vi "Galobal variable_TI.vi"() -> ()   [LabVIEW 2015]
panel:
  in  "Operator ID":string="OB"
  in  "Server":bool
  in  "Shift":T1
  in  "Rework bit":bool
  in  "NG Count":u8
  in  "Shift  Change":string
  in  "User ID":string="OB"
  out "Emergency Analog":bool
  out "Errror For Color":bool
  in  "Pokayoka Status":bool
  in  "Rpt Write 2":bool
  in  "Rpt Write":bool
  in  "Rpt Read":bool
  in  "Model triger":bool
  in  "Camera Bit":string
  out "Error Color":u32
  in  "Cali data":T2
  out "Camera NG":bool
  in  "CAMERA TRIGGER":bool
  out "Camera OK":bool
  out "Cordinate":string
  in  "LCD  Barcode_Trigger":bool
  in  "MIC Barcode _Trigger":bool
  in  "MIC Barcode":string
  in  "LCD Barcode":string
  in  "Barcode Setting":T3={"MIC "="", "baud rate MIC "=9600, "LCD "="COM5", "baud rate_LCD"=115200}
  out "IL Sensor_Pokayoka":bool[](array[boolean])
  in  "Running Model":string
  in  "Sensor Setting Data":T4
  out "Sensor Data":T5
  in  "NI Comm.Error":bool
  in  "LVDT":dbl format="%0.03f"
  in  "Load Cell":dbl format="%0.03f"
  in  "Digital Output":bool[](array[boolean])
  in  "Auto Exit":bool
  in  "Slid Servo Home bit":bool
  in  "Call Home M2":bool
  in  "Call Home M1":bool
  in  "Barcode Lenght":i32
  in  "Barcode Scan Bit":bool
  in  "Barcode Data":string
  in  "Control Enable":bool
  in  "Stop M1":bool
  in  "Stop M2":bool
  in  "Programlist":string[](array[string])
  in  "STM Done Bit":bool
  in  "Offset_2":dbl
  in  "Offset_1":dbl
  in  "Slop _2":dbl
  in  "Slop_1":dbl
  out "Analoge Input":dbl[](array[numeric])
  out "AI_as DI":bool[](array[boolean])
  out "Manual DO":bool[](array[boolean])
  in  "Manual CMD":bool
  out "File Path":path[](array[path])
  out "Digital input":bool[](array[boolean])
  in  "User Name":string
  in  "Exit":bool
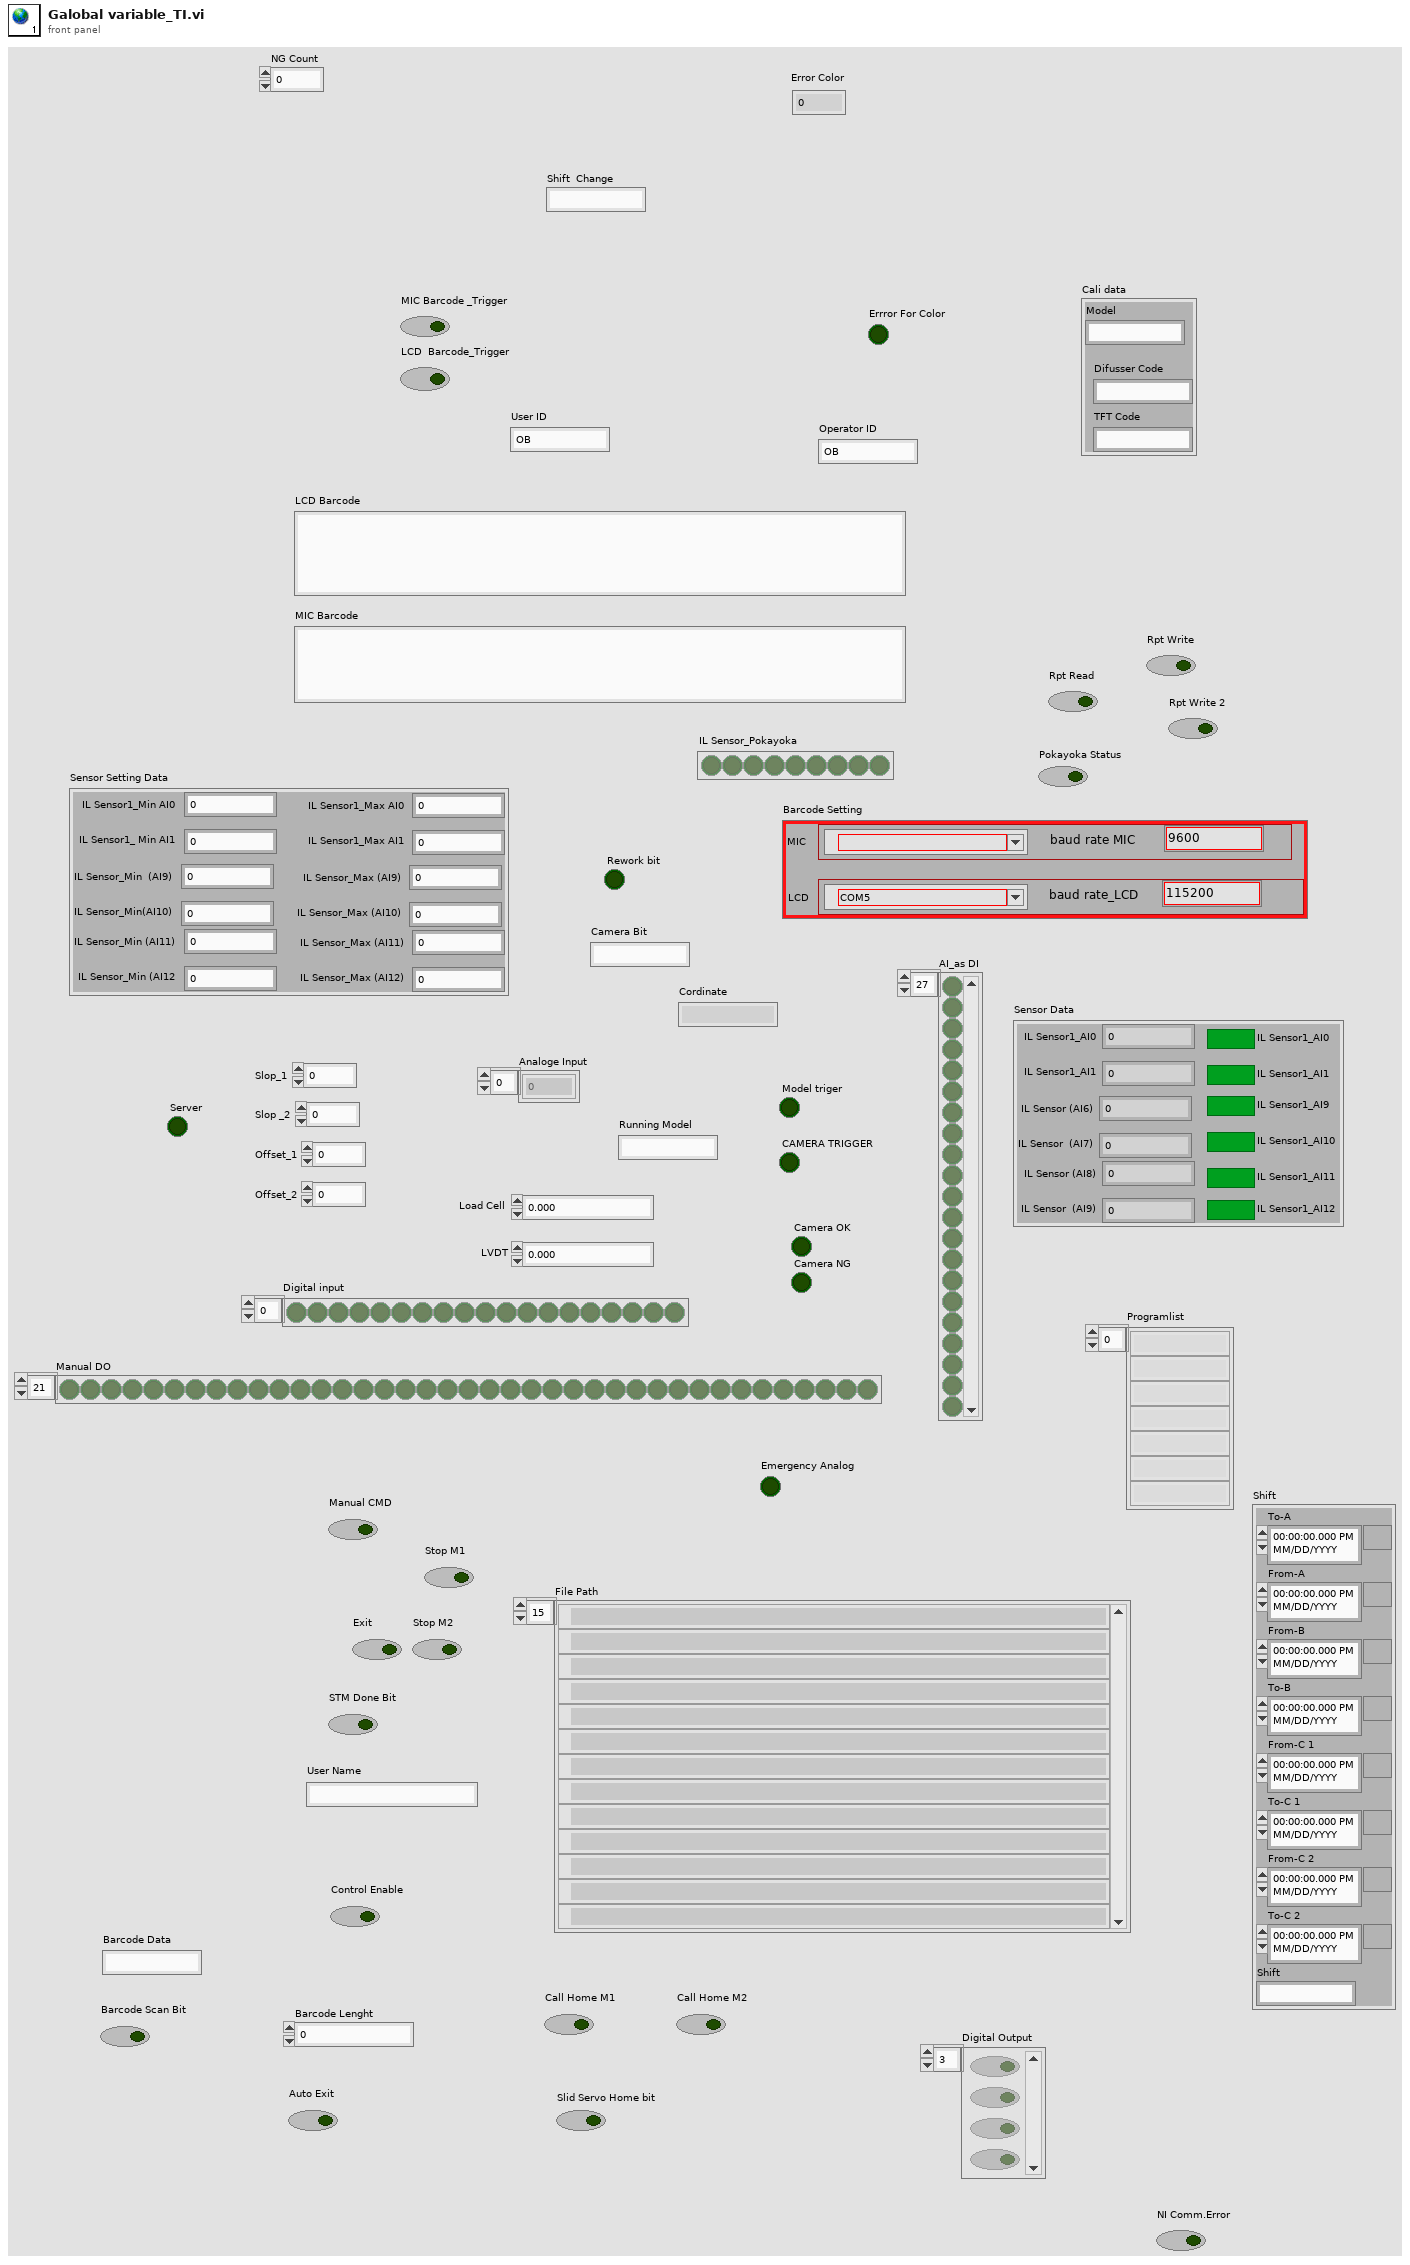
[diagram p1: front panel]
types:
  T1 = cluster{"To-A":timestamp, "From-A":timestamp, "From-B":timestamp, "To-B":timestamp, "From-C 1":timestamp, "To-C 1":timestamp, "From-C 2":timestamp, "To-C 2":timestamp, "Shift":string}
  T2 = cluster{"Model":string, "Difusser Code":string, "TFT Code ":string}
  T3 = cluster{"MIC ":refnum<visa-resource-name>, "baud rate MIC ":u32, "LCD ":refnum<visa-resource-name>, "baud rate_LCD":u32}
  T4 = cluster{"IL Sensor1_Max AI0":dbl, "IL Sensor1_Min AI0":dbl, "IL Sensor1_Max AI1":dbl, "IL Sensor1_ Min AI1":dbl, "IL Sensor_Max (AI9)":dbl, "IL Sensor_Min  (AI9)":dbl, "IL Sensor_Max (AI10)":dbl, "IL Sensor_Min(AI10)":dbl, "IL Sensor_Max (AI11)":dbl, "IL Sensor_Min (AI11)":dbl, "IL Sensor_Max (AI12)":dbl, "IL Sensor_Min (AI12":dbl}
  T5 = cluster{"IL Sensor1_AI0":dbl, "IL Sensor1_AI1":dbl, "IL Sensor (AI6)":dbl, "IL Sensor  (AI7)":dbl, "IL Sensor (AI8)":dbl, "IL Sensor  (AI9)":dbl, "IL Sensor1_AI0":bool, "IL Sensor1_AI1":bool, "IL Sensor1_AI9":bool, "IL Sensor1_AI10":bool, "IL Sensor1_AI11":bool, "IL Sensor1_AI12":bool}
diagram:
